vi "create_from_existing.vi"(10 "dataset RID":string) -> (3 "Existing Target":refnum<class "target.lvclass">)   [LabVIEW 2020, in "datasources.lvlib" / "target.lvclass"]
uses:
  target.lvclass
  dataset/dataset.lvclass
  dataset/dataset.lvclass/dataset.ctl
  target.lvclass/target.ctl
  dataset/rid.set.vi
  dataset.set.vi
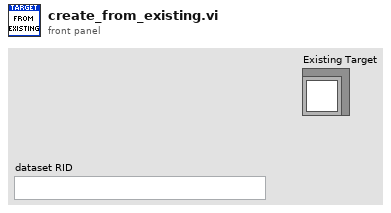
[diagram p1: front panel]
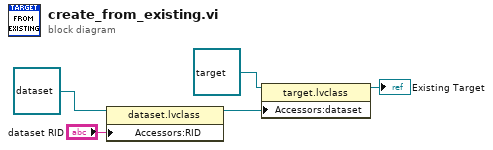
[diagram p0: block diagram]
diagram:
  n1 = property class="dataset.lvclass"(reference=refnum<class "dataset.lvclass"> refnum ("datasources.lvlib:dataset.lvclass"), "Accessors:RID"="dataset RID") -> (reference out=w2:refnum<class "dataset.lvclass">)  [unwired: 1 in, 1 out]
  n2 = property class="target.lvclass"(reference=refnum<class "target.lvclass"> refnum ("Target"), "Accessors:dataset"=w2) -> (reference out=→"Existing Target":refnum<class "target.lvclass">)  [unwired: 1 in, 1 out]
